vi "Output Quantities.vi"() -> ()   [LabVIEW 2013]
uses:
  qwtblvlib/TD Quantity.ctl
  <vilib>/Math Plots/2D Math Plots/2D Error Bar/2D Error Bar XCtrl/2D Error Bar.xctl
  <vilib>/Math Plots/3D Math Plots/3D Surface/3D Surface XCtrl/3D Surface.xctl
  globals.vi
  <vilib>/gmath/interp.llb/Create Mesh Grid (2D) (x,y arrays).vi
  <vilib>/Math Plots/3D Math Plots/3D Surface/3D Surface Datatype/Public/Plot Helper (Matrix).vi
  <vilib>/Math Plots/2D Math Plots/2D Error Bar/2D Error Bar Datatype/Public/Plot Helper (Fixed).vi
  <vilib>/Analysis/NI_AALBase.lvlib
  <vilib>/Math Plots/2D Math Plots/2D Error Bar/2D Error Bar Datatype/2D Error Bar Datatype.lvclass
  <vilib>/Math Plots/3D Math Plots/3D Surface/3D Surface Datatype/3D Surface Datatype.lvclass
  <vilib>/gmath/NI_Gmath.lvlib
  qwtblvlib/QWTBLVLib.lvlib
panel:
  in  "hide this panel":bool
  in  "redraw quantity signal":bool
  in  "Qtab":enum32{"Value/Graph", "Histogram", "Raw values"}(tab)
  out "value 3D":refnum<class "3D Plot Datatype.lvclass">[](xcontrol)
  out "value 2D":refnum<class "2D Plot Datatype.lvclass">[](xcontrol)
  out "value string":string
  out "Histogram Graph":T1(graph)
  out "hist-notOK":string
  out "Selected Quantity":T2={"Name"="", "Value"=[[1.0]], "Uncertainty"=[[1.0]], "Degrees of Freedom"=[[10.0]], "Correlation"=[[10.0]], "Randomized uncertainty"=[[10.0]]}
  in  "new data signal":bool
  in  "Q list":i32(listbox) caption="List of\noutput Quantities"
  # "Output Quantities"
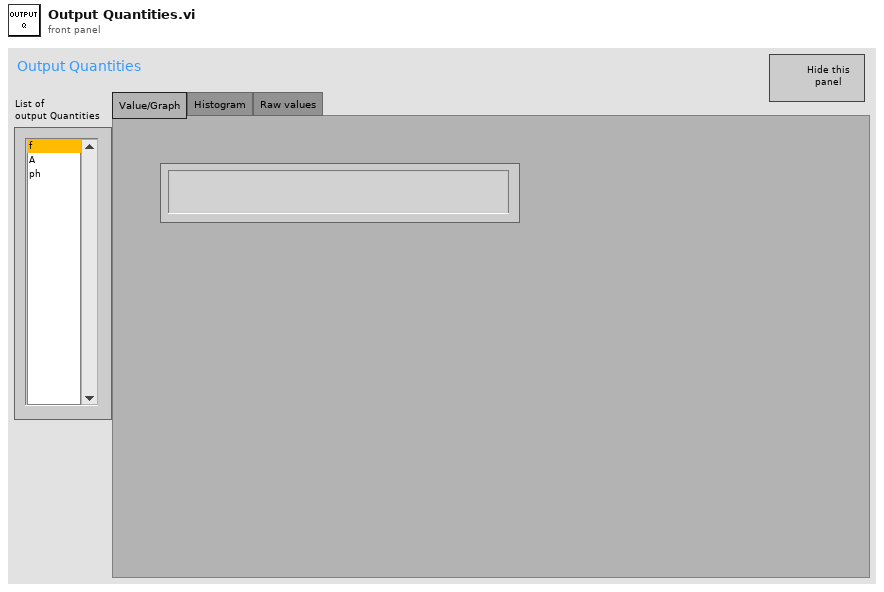
[diagram p1: front panel]
types:
  T1 = cluster{"X Values":dbl[], "Histogram: h(x)":i32[]}
  T2 = typedef "QWTBLVLib.lvlib/TD Quantity.ctl" = cluster{"Name":string, "Value":dbl[][], "Uncertainty":dbl[][], "Degrees of Freedom":dbl[][], "Correlation":dbl[][], "Randomized uncertainty":dbl[][]}
  T3 = enum32{"Invalid", "Standard", "Closed", "Hidden", "Minimized", "Maximized"}
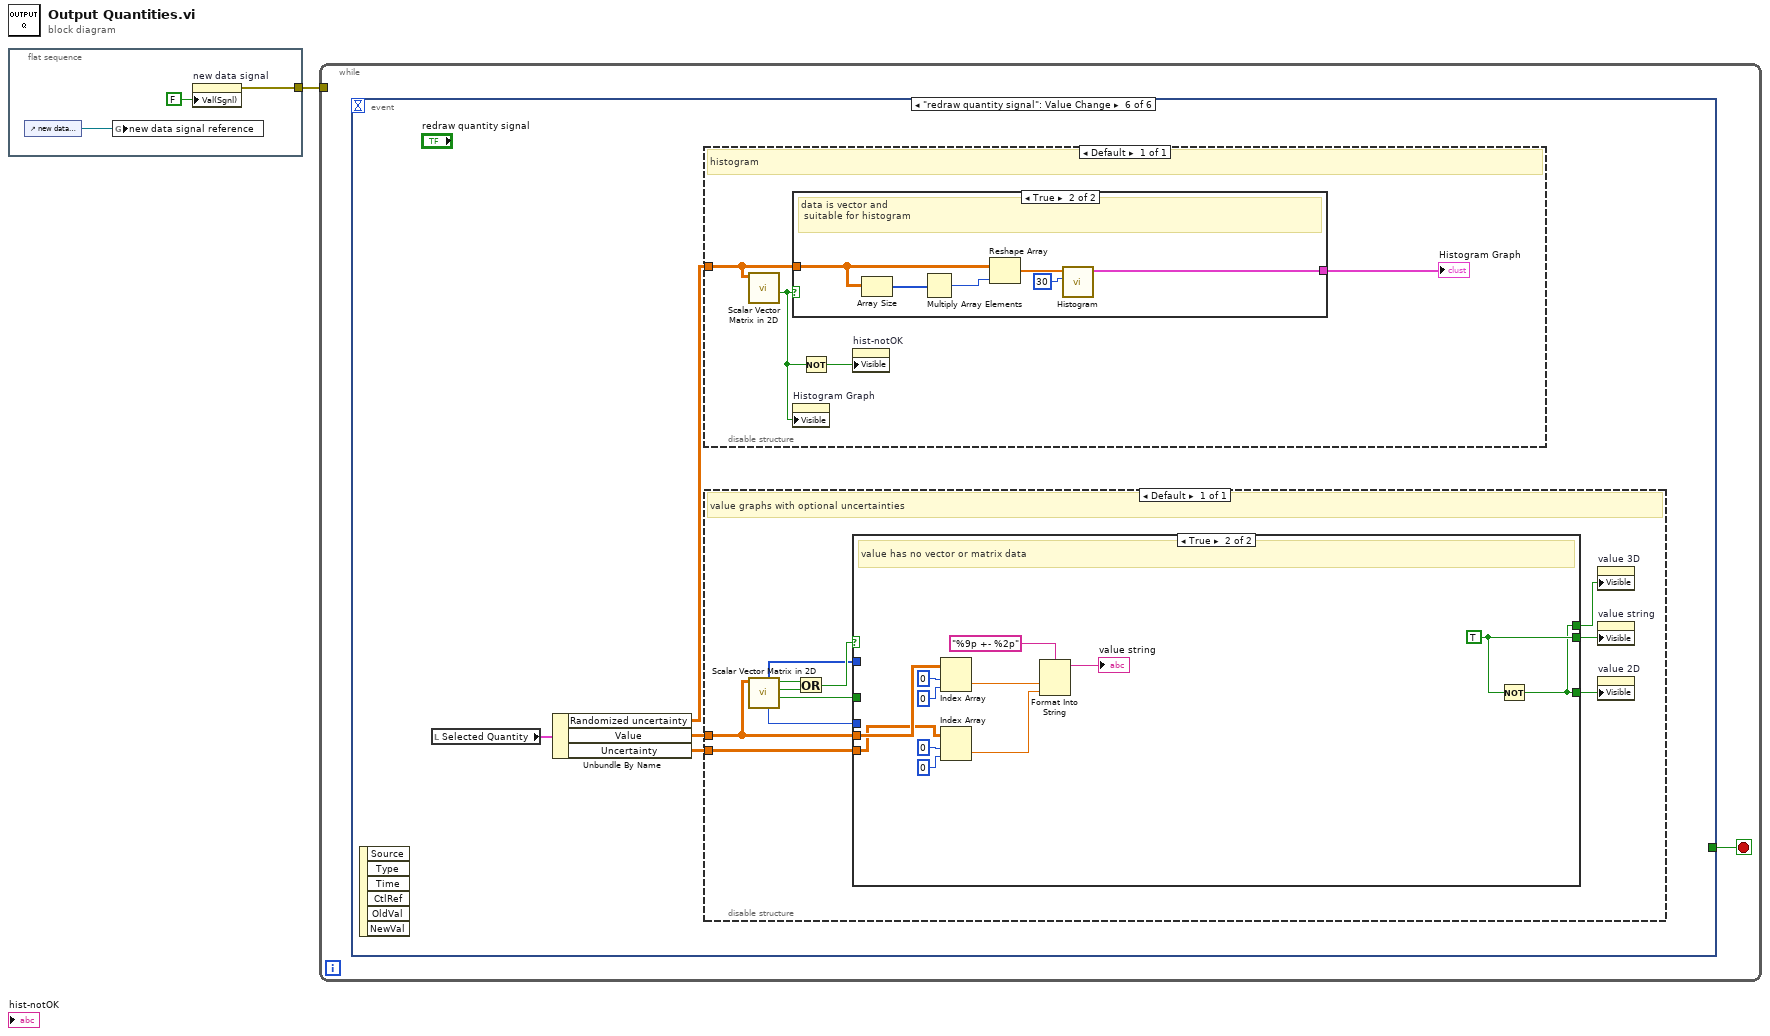
[diagram p0: block diagram]
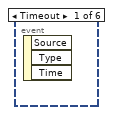
[diagram p2: hidden frame]
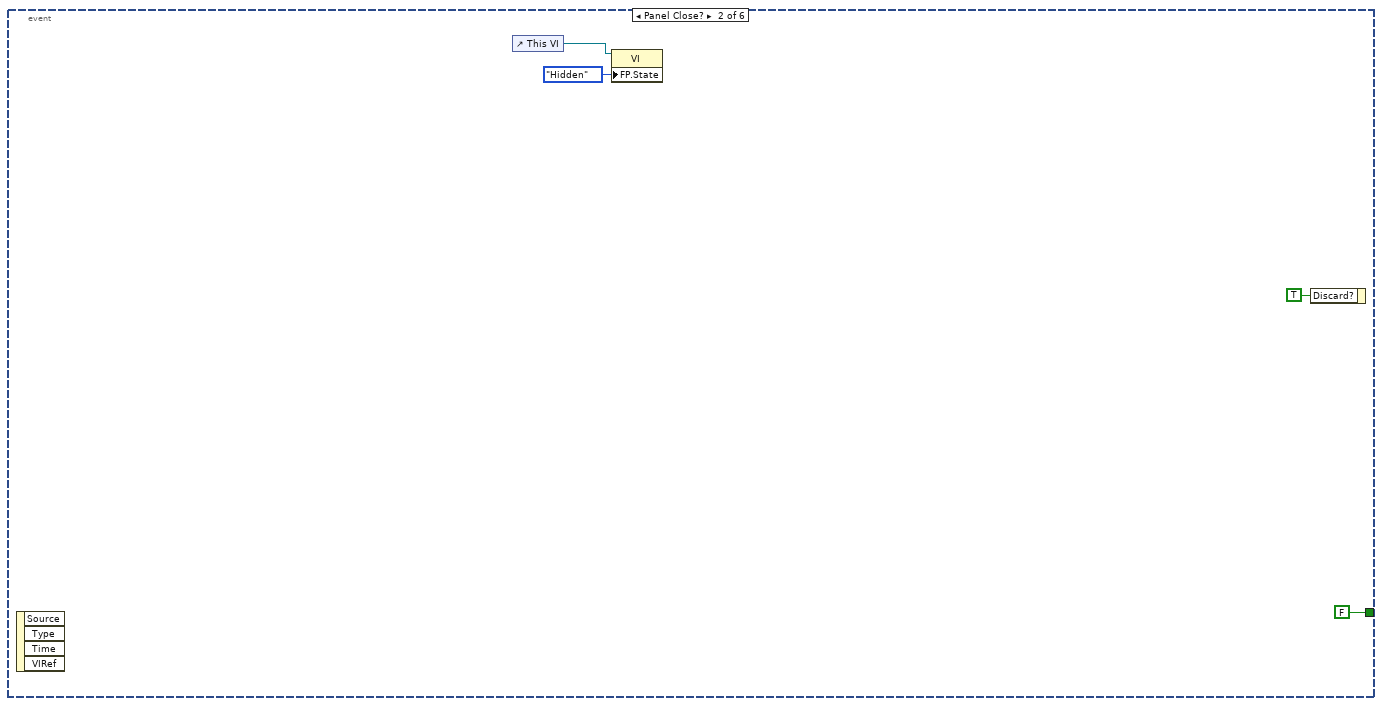
[diagram p3: hidden frame]
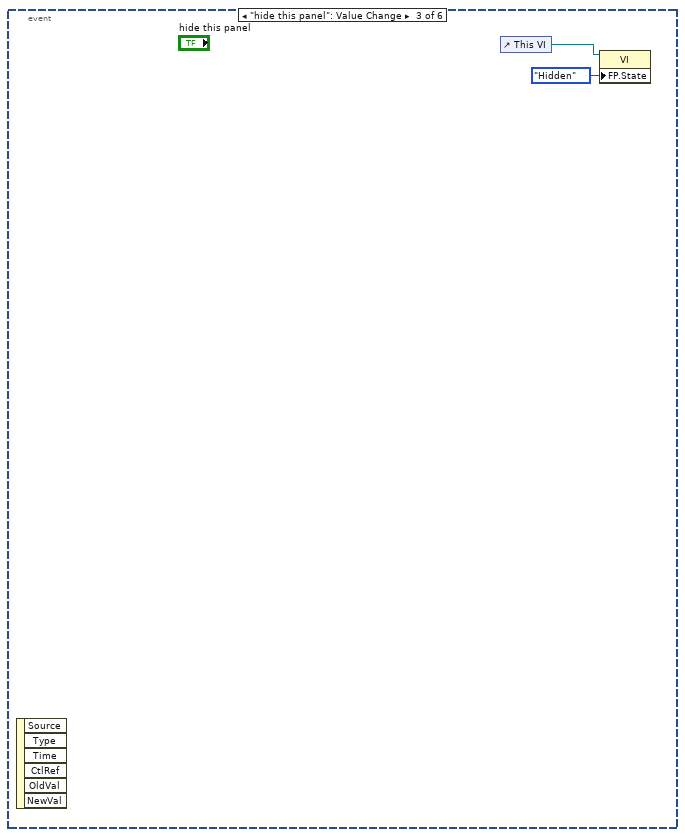
[diagram p4: hidden frame]
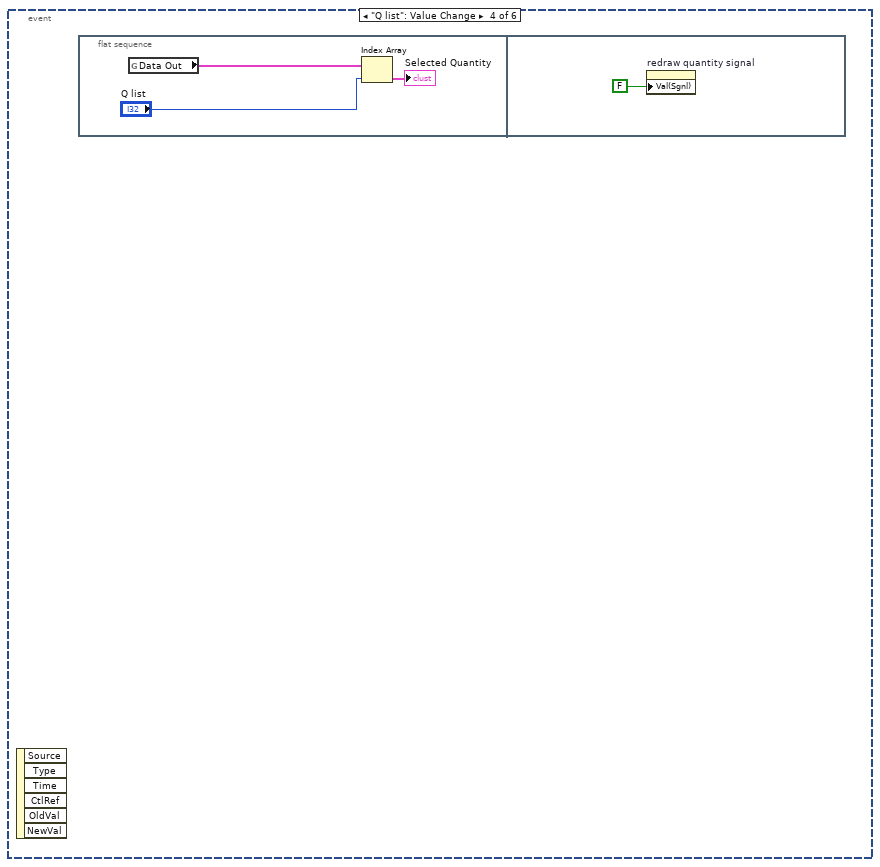
[diagram p5: hidden frame]
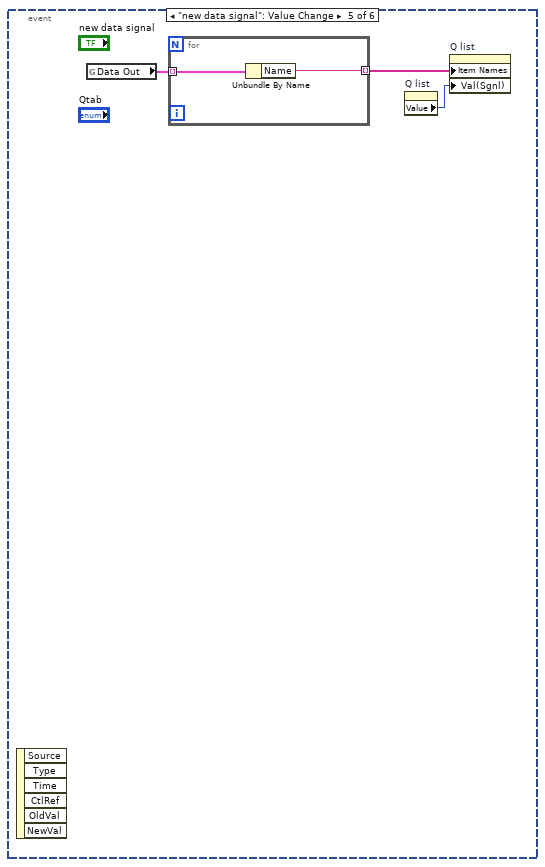
[diagram p6: hidden frame]
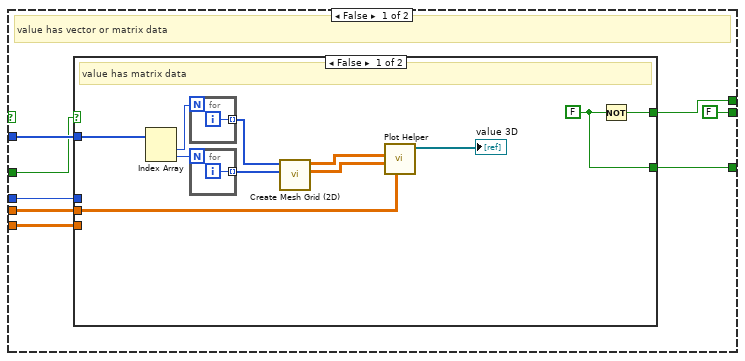
[diagram p7: hidden frame]
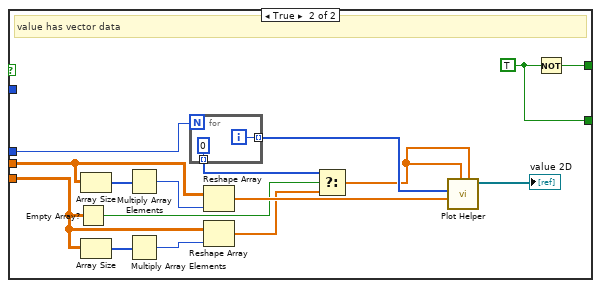
[diagram p8: hidden frame]
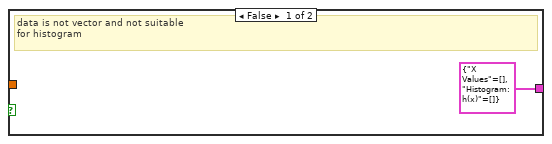
[diagram p9: hidden frame]
diagram:
  n1 = flat-sequence {
    tunnel: [w2] -> w1
    frame #0 {
      n2 = control-ref of="new data signal"() -> (w4:refnum<vi>)
      n3 = global write "globals.vi" "new data signal reference"(w4) -> ()
      n4 = property on="new data signal" class="Bool (strict)"("Val(Sgnl)"=FALSE ("Value (Signaling)")) -> (error out=w2:errorcluster)  [unwired: 2 in, 1 out]
    }
  }
  n5 = while {
    tunnel: w1 -> [_]
    stop <- w5 stop-if-true
    n6 = event shown="[5] \"redraw quantity signal\": Value Change" {
      selector: _ -> [_ _ _ _ _ _]
      dyn-events: _ -> [_ _ _ _ _ _]
      timeout: _ -> [_ _ _ _ _ _]
      tunnel: [_ FALSE _ _ _ _] -> w5
      event Timeout {
        n7 = event-data() -> ()  [unwired: 1 in, 3 out]
      }
      event Panel Close? {
        n8 = event-data() -> ()  [unwired: 1 in, 4 out]
        n9 = control-ref of="This VI"() -> (w7:refnum<vi>)
        n10 = property class="VI"(reference=w7, "FP.State"=T3."Hidden" ("Front Panel Window:State")) -> ()  [unwired: 1 in, 2 out]
        n11 = event-data("Discard?"=TRUE) -> ()  [unwired: 1 in, 1 out]
      }
      event "hide this panel": Value Change {
        n12 = event-data() -> ()  [unwired: 1 in, 6 out]
        n13 = control-ref of="This VI"() -> (w11:refnum<vi>)
        n14 = property class="VI"(reference=w11, "FP.State"=T3."Hidden" ("Front Panel Window:State")) -> ()  [unwired: 1 in, 2 out]
      }
      event "Q list": Value Change {
        n15 = event-data() -> ()  [unwired: 1 in, 6 out]
        n16 = flat-sequence {
          frame #0 {
            n17 = global read "globals.vi" "Data Out"() -> (w14:T2[])
            n18 = Index Array(array=w14, index="Q list") -> (element=→"Selected Quantity":T2)
          }
          frame #1 {
            n19 = property on="redraw quantity signal" class="Bool (strict)"("Val(Sgnl)"=FALSE ("Value (Signaling)")) -> ()  [unwired: 2 in, 2 out]
          }
        }
      }
      event "new data signal": Value Change {
        n20 = event-data() -> ()  [unwired: 1 in, 6 out]
        n21 = global read "globals.vi" "Data Out"() -> (w18:T2[])
        n22 = for {
          tunnel: [w20] -> w17 mode=indexing
          tunnel: w18 -> [w19] mode=indexing
          n23 = Unbundle By Name(w19) -> ("Name"=w20:string)
        }
        n24 = property on="Q list" class="LstBox (strict)"() -> ("Value"=w16:i32)  [unwired: 2 in, 2 out]
        n25 = property on="Q list" class="LstBox (strict)"("Item Names"=w17, "Val(Sgnl)"=w16) -> ()  [unwired: 2 in, 2 out]
      }
      event "redraw quantity signal": Value Change {
        n26 = event-data() -> ()  [unwired: 1 in, 6 out]
        n27 = local read "Selected Quantity"() -> (w24:T2)
        n28 = Unbundle By Name(w24) -> ("Randomized uncertainty"=w23:dbl[][], "Value"=w22:dbl[][], "Uncertainty"=w21:dbl[][])
        n29 = disable-structure shown="Default" {
          disable-tunnel: w23 -> [w88]
          frame Enabled {
            # "histogram"
            n30 = call "Scalar Vector Matrix in 2D.vi"("2D Array"=w88) -> ("Is Vector?"=w87:bool)  [unwired: 4 in, 6 out]
            n31 = case shown="True" w87 {
              tunnel: [T1 {"X Values"=[], "Histogram: h(x)"=[]} ("Histogram Graph") w97] -> w89
              tunnel: w88 -> [_ w93]
              frame False {
                # "data is not vector and not suitable\nfor histogram"
              }
              frame True {
                # "data is vector and\n suitable for histogram"
                n32 = Array Size(array=w93) -> (size(s)=w94:i32[])
                n33 = Multiply Array Elements(1:w94) -> (0:w92:i32)
                n34 = Reshape Array(w93, w92) -> (w95:dbl[])
                n35 = call <vilib>:"Histogram.vi"("intervals"=30, "X"=w95) -> ("Histogram Graph"=w97:T1)  [unwired: 6 in, 3 out]
              }
            }
            "Histogram Graph" <- w89
            n36 = property on="Histogram Graph" class="XYGraph (strict)"("Visible"=w87) -> ()  [unwired: 2 in, 2 out]
            n37 = Not(x=w87) -> (.not. x?=w90:bool)
            n38 = property on="hist-notOK" class="Str"("Visible"=w90) -> ()  [unwired: 2 in, 2 out]
          }
        }
        n39 = disable-structure shown="Default" {
          disable-tunnel: w22 -> [w32]
          disable-tunnel: w21 -> [w31]
          frame Enabled {
            # "value graphs with optional uncertainties"
            n40 = call "Scalar Vector Matrix in 2D.vi"("2D Array"=w32) -> ("Is Vector?"=w27:bool, "Is Scalar?"=w29:bool, "Is Empty?"=w30:bool, "Dim Max"=w26:i32, "Dimensions"=w25:i32[])  [unwired: 4 in, 2 out]
            n41 = Or(x=w30, y=w29) -> (x .or. y?=w28:bool)
            n42 = case shown="True" w28 {
              tunnel: [FALSE ("Visible") w86] -> w35
              tunnel: [w41 w85] -> w34
              tunnel: [w42 w85] -> w33
              tunnel: w32 -> [w40 w78]
              tunnel: w25 -> [w39 _]
              tunnel: w31 -> [w38 w75]
              tunnel: w27 -> [w37 _]
              tunnel: w26 -> [w36 _]
              frame False {
                # "value has vector or matrix data"
                n43 = case shown="False" w37 {
                  tunnel: [w53 w62] -> w42
                  tunnel: [w54 w63] -> w41
                  tunnel: w40 -> [w51 w68]
                  tunnel: w39 -> [w48 _]
                  tunnel: w36 -> [_ w70]
                  tunnel: w38 -> [_ w61]
                  frame False {
                    w53 = FALSE ("Visible")
                    # "value has matrix data"
                    n44 = Index Array(array=w48) -> (element #1=w44:i32, element #2=w47:i32)  [unwired: 2 in]
                    n45 = for {
                      N: w44 -> [_]
                      tunnel: [w55] -> w45 mode=indexing
                      i -> [w55]
                    }
                    n46 = for {
                      N: w47 -> [_]
                      tunnel: [w56] -> w46 mode=indexing
                      i -> [w56]
                    }
                    n47 = call-poly <vilib>:"Create Mesh Grid (2D).vi"("y domain"=w46, "x domain"=w45) -> ("Y"=w49:dbl[][], "X"=w50:dbl[][])  [unwired: 7 in, 1 out]
                    n48 = call-poly <vilib>:"Plot Helper.vi"("z matrix"=w51, "y matrix"=w49, "x matrix"=w50) -> ("3D Plot lvclass Array out"=→"value 3D":refnum<class "3D Plot Datatype.lvclass">[])  [unwired: 3 in, 5 out]
                    n49 = Not(x=w53) -> (.not. x?=w54:bool)
                  }
                  frame True {
                    w62 = TRUE ("Visible")
                    # "value has vector data"
                    n50 = Empty Array?(array=w61) -> (empty?=w60:bool)
                    n51 = Array Size(array=w68) -> (size(s)=w67:i32[])
                    n52 = Array Size(array=w61) -> (size(s)=w65:i32[])
                    n53 = Multiply Array Elements(1:w67) -> (0:w66:i32)
                    n54 = Multiply Array Elements(1:w65) -> (0:w64:i32)
                    n55 = for {
                      N: w70 -> [_]
                      tunnel: [w74] -> w69 mode=indexing
                      tunnel: [0 ("product")] -> w59 mode=indexing
                      i -> [w74]
                    }
                    n56 = Reshape Array(w68, w66) -> (w71:dbl[])
                    n57 = Reshape Array(w61, w64) -> (w58:dbl[])
                    n58 = Select(t=w59, s=w60, f=w58) -> (s? t:f=w57:dbl[])
                    n59 = call-poly <vilib>:"Plot Helper.vi"("error b vector"=w57, "error a vector"=w57, "y vector"=w71, "x vector"=w69) -> ("2D Plot Class Obj Array out"=→"value 2D":refnum<class "2D Plot Datatype.lvclass">[])  [unwired: 2 in, 5 out]
                    n60 = Not(x=w62) -> (.not. x?=w63:bool)
                  }
                }
              }
              frame True {
                w86 = TRUE ("Visible")
                # "value has no vector or matrix data"
                n61 = Index Array(array=w78, index (row)=0, index (col)=0 ("disabled index (col)")) -> (element=w81:dbl)
                n62 = Index Array(array=w75, index (row)=0, index (col)=0 ("disabled index (col)")) -> (element=w77:dbl)
                n63 = Format Into String(format string="%9p +- %2p", w81, w77) -> (resulting string=→"value string":string)  [unwired: 2 in, 1 out]
                n64 = Not(x=w86) -> (.not. x?=w85:bool)
              }
            }
            n65 = property on="value 3D" class="3D Surface (strict)"("Visible"=w34) -> ()  [unwired: 2 in, 2 out]
            n66 = property on="value string" class="Str"("Visible"=w35) -> ()  [unwired: 2 in, 2 out]
            n67 = property on="value 2D" class="2D Error Bar (strict)"("Visible"=w33) -> ()  [unwired: 2 in, 2 out]
          }
        }
      }
    }
  }
